vi "NI Switch Single Connect.vi"(8 "error in (no error)":errorcluster, 9 "channel 2":string, 10 "channel 1":string, 11 "RelayOutput in":refnum<class "NISwitch.lvclass">) -> (0 "error out":errorcluster, 3 "RelayOutput out":refnum<class "NISwitch.lvclass">)   [LabVIEW 2023, in "HardwareAbstractionLayer_LVOOP.lvlib" / "NISwitch.lvclass"]
uses:
  NISwitch.lvclass
  NISwitch.lvclass/NISwitch.ctl
  <instrlib>/niSwitch/niSwitch.llb/niSwitch Connect Channels (Single).vi
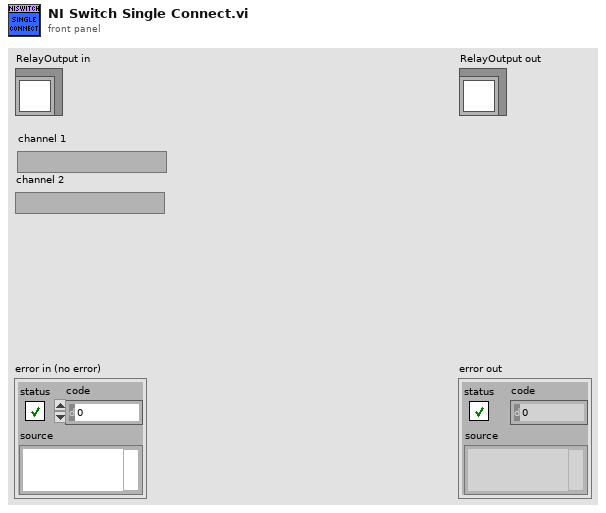
[diagram p1: front panel]
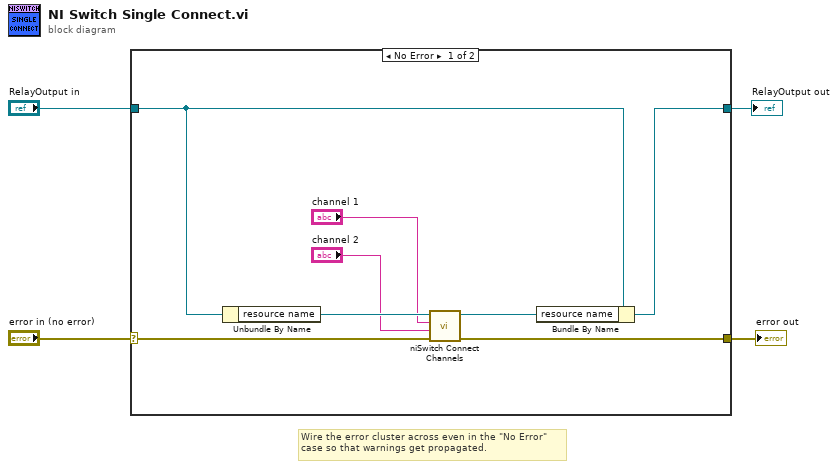
[diagram p0: block diagram]
diagram:
  # "Wire the error cluster across even in the \"No Error\"\ncase so that warnings get propagated."
  n1 = case shown="No Error" "error in (no error)" {
    selector: "error in (no error)" -> [w11 w14]
    tunnel: [w10 w14] -> w3
    tunnel: [w8 w13] -> w1
    tunnel: "RelayOutput in" -> [w9 w13]
    frame No Error {
      n2 = Unbundle By Name(w9) -> ("resource name"=w12:refnum<k15>)
      n3 = call-poly <instrlib>:"niSwitch Connect Channels.vi"("error in (no error)"=w11, "channel 2"="channel 2", "channel 1"="channel 1", "instrument handle"=w12) -> ("error out"=w10:errorcluster, "instrument handle out"=w7:refnum<k15>)  [unwired: 6 in]
      n4 = Bundle By Name(cluster=w9, "resource name"=w7) -> (w8:refnum<class "NISwitch.lvclass">)
    }
    frame Error {
    }
  }
  "error out" <- w3
  "RelayOutput out" <- w1
